vi "TargetCoord.vi"(3 "CenterXIn":dbl, 4 "CenterYIn":dbl, 5 "ScoreIn":dbl, 7 "MinScore":dbl, 9 "Update?":bool) -> (17 "CenterXOut":dbl, 18 "CenterYOut":dbl, 19 "Target?":bool)   [LabVIEW 2016]
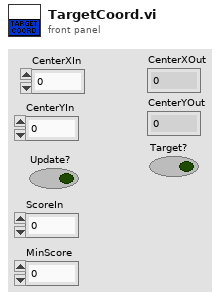
[diagram p1: front panel]
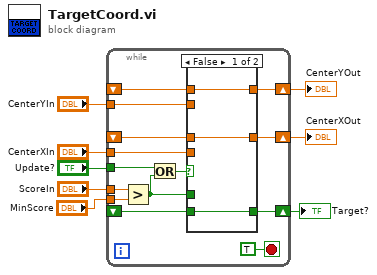
[diagram p0: block diagram]
diagram:
  n1 = while {
    shift-right: [w18] -> w8
    shift-left: _ -> [w19]
    shift-right: [w20] -> w7
    shift-left: _ -> [w21]
    tunnel: "CenterYIn" -> [w16]
    tunnel: "CenterXIn" -> [w17]
    tunnel: "Update?" -> [w12]
    tunnel: "ScoreIn" -> [w11]
    shift-right: [w15] -> w2
    shift-left: _ -> [w14]
    tunnel: "MinScore" -> [w9]
    stop <- TRUE stop-if-true
    n2 = Greater?(x=w11, y=w9) -> (0:w10:bool)
    n3 = Or(x=w12, y=w10) -> (x .or. y?=w13:bool)
    n4 = case shown="False" w13 {
      tunnel: w21 -> [w25 _]
      tunnel: [w25 w27] -> w20
      tunnel: w19 -> [w24 _]
      tunnel: [w24 w28] -> w18
      tunnel: w17 -> [_ w28]
      tunnel: w16 -> [_ w27]
      tunnel: w10 -> [_ w26]
      tunnel: [w23 w26] -> w15
      tunnel: w14 -> [w23 _]
      frame False {
      }
      frame True {
      }
    }
  }
  "CenterXOut" <- w8
  "CenterYOut" <- w7
  "Target?" <- w2
